vi "EX 10-2_TempControl.vi"() -> ()   [LabVIEW 2010]
uses:
  <vilib>/LabVIEW Interface for Arduino/Type Defs/Pin Mode.ctl
  <vilib>/LabVIEW Interface for Arduino/Type Defs/Board Type.ctl
  <vilib>/LabVIEW Interface for Arduino/Type Defs/Connection Type.ctl
  <vilib>/LabVIEW Interface for Arduino/LabVIEW Interface for Arduino.lvlib
panel:
  in  "手動     /    自動":bool
  in  "熱敏電阻PIN腳":u8
  in  "Units":enum16{"Celsius", "Fahrenheit", "Kelvin"}(ring)
  out "Temperature":dbl(slide) scale=0.0..100.0
  in  "Paired Resistance (Ohms)":dbl=10000.0
  in  "motor 3":u8(slide) scale=0.0..255.0
  in  "motor 1":u8(slide) scale=0.0..255.0
  in  "motor 2":u8(slide) scale=0.0..255.0
  in  "Heater":bool
  in  "最高溫度":dbl
  in  "最低溫度":dbl
  in  "stop":bool
  in  "風扇3 PIN腳":u8=6 min=2 max=13 step=1
  in  "風扇2 PIN腳":u8=5 min=2 max=13 step=1
  in  "風扇1 PIN腳":u8=3 min=2 max=13 step=1
  in  "加熱片PIN腳":u8
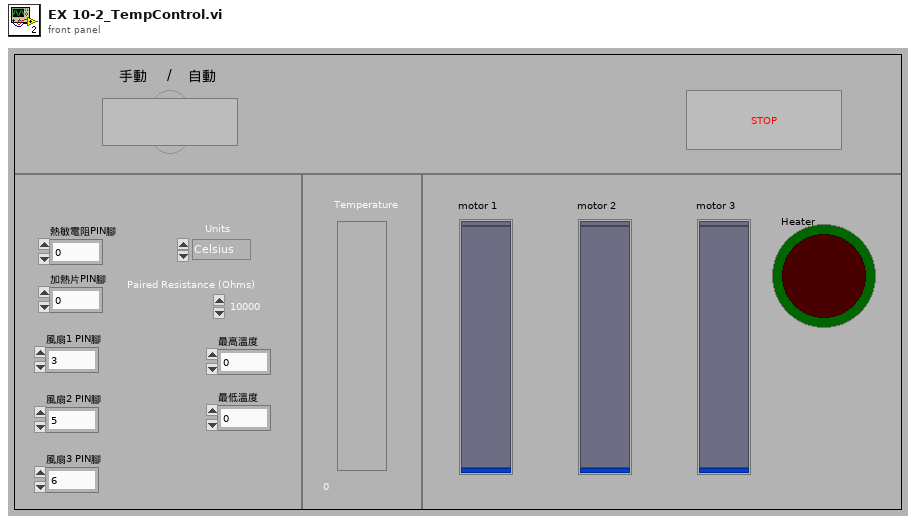
[diagram p1: front panel]
types:
  T1 = typedef "LabVIEW Interface for Arduino.lvlib/Connection Type.ctl" = enum8{"USB / Serial", "XBEE", "BlueSmirf (Bluetooth)"}
  T2 = typedef "LabVIEW Interface for Arduino.lvlib/Board Type.ctl" = enum16{"Uno", "Dimuelanove w/Atmega 328", "Mega 2560"}
  T3 = typedef "LabVIEW Interface for Arduino.lvlib/Pin Mode.ctl" = enum8{"Input", "Output"}
  T4 = typedef "LabVIEW Interface for Arduino.lvlib/Arduino Resource.ctl" = cluster{"VISA resource":refnum<visa-resource-name>, "Board Type":T2, "Connection Type":enum8{"USB / Serial"}, "Bytes Per Packet (15)":u8}
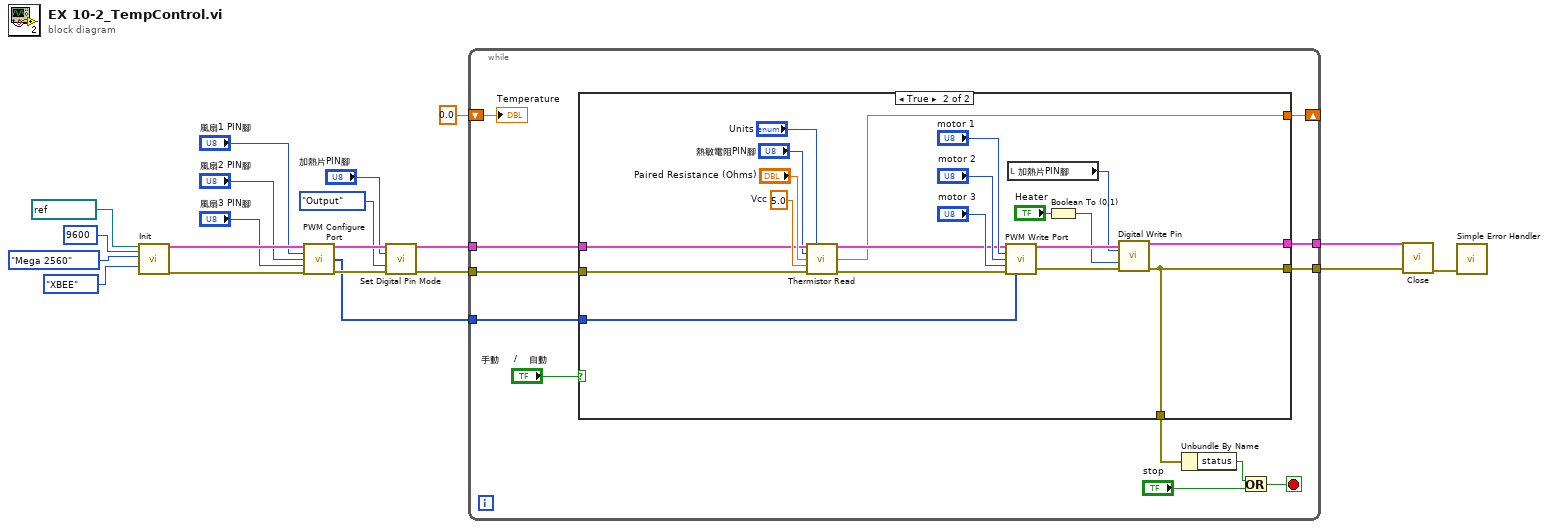
[diagram p0: block diagram]
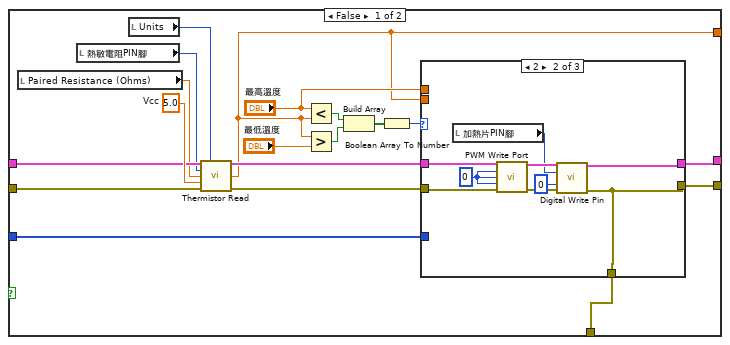
[diagram p2: hidden frame]
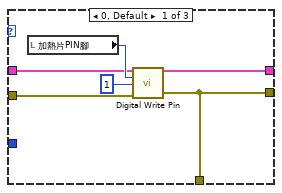
[diagram p3: hidden frame]
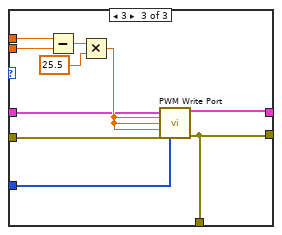
[diagram p4: hidden frame]
diagram:
  n1 = call <vilib>:"Init.vi"("VISA resource"=refnum<visa-resource-name> "COM8", "Baud Rate (115200)"=u32 9600, "Board Type (Uno)"=Board_Type."Mega 2560", "Connection Type (USB/Serial)"=Connection_Type."XBEE") -> ("Arduino Resource"=w19:T4, "error out"=w18:errorcluster)  [unwired: 14 in]
  n2 = call <vilib>:"PWM Configure Port.vi"("Arduino Resource"=w19, "PWM Pin (3)"="風扇1 PIN腳", "PWM Pin (5)"="風扇2 PIN腳", "PWM Pin (6)"="風扇3 PIN腳", "error in"=w18) -> ("Arduino Resource"=w14:T4, "PWM Pins"=w2:u8[], "error out"=w13:errorcluster)  [unwired: 8 in]
  n3 = call <vilib>:"Set Digital Pin Mode.vi"("Arduino Resource"=w14, "Digital I/O Pin"="加熱片PIN腳", "Pin Mode (Input)"=Pin_Mode."Output", "error in"=w13) -> ("Arduino Resource"=w10:T4, "error out"=w9:errorcluster)  [unwired: 10 in]
  n4 = while {
    tunnel: w10 -> [w31]
    tunnel: w9 -> [w30]
    tunnel: [w29] -> w8
    tunnel: [w28] -> w7
    tunnel: w2 -> [w23]
    shift-right: [w21] -> _
    shift-left: 0.0 ("Temperature") -> [w22]
    stop <- w24 stop-if-true
    n5 = case shown="True" "手動     /    自動" {
      tunnel: w31 -> [w50 w93]
      tunnel: w30 -> [w49 w92]
      tunnel: [w38 w80] -> w29
      tunnel: [w36 w79] -> w27
      tunnel: [w37 w79] -> w28
      tunnel: w23 -> [w35 w78]
      tunnel: [w33 w77] -> w21
      frame False {
        w51 = 5.0  # Vcc
        n6 = local read "Paired Resistance (Ohms)"() -> (w46:dbl)
        n7 = local read "熱敏電阻PIN腳"() -> (w47:u8)
        n8 = local read "Units"() -> (w48:enum16{"Celsius", "Fahrenheit", "Kelvin"})
        n9 = call <vilib>:"Thermistor Read.vi"("Arduino Resource"=w50, "Units (C)"=w48, "Thermistor AI Pin (0)"=w47, "Paired Resistance (10K Ohms)"=w46, "Vcc (5 v)"=w51, "error in"=w49) -> ("Arduino Resource"=w40:T4, "Temperature"=w33:dbl, "error out"=w39:errorcluster)  [unwired: 7 in]
        n10 = Less?(x="最高溫度", y=w33) -> (x < y?=w44:bool)
        n11 = Greater?(x=w33, y="最低溫度") -> (0:w43:bool)
        n12 = Build Array(w44, w43) -> (w42:bool[])
        n13 = Boolean Array To Number(Boolean array=w42) -> (number=w41:u32)
        n14 = case shown="2" w41 {
          tunnel: w40 -> [w55 w61 w73]
          tunnel: w39 -> [w54 w60 w72]
          tunnel: [w53 w59 w71] -> w38
          tunnel: [w52 w58 w67] -> w37
          tunnel: [w52 w58 w67] -> w36
          tunnel: w35 -> [_ _ w70]
          tunnel: "最高溫度" -> [_ _ w69]
          tunnel: w33 -> [_ _ w68]
          frame 0, Default {
            n15 = local read "加熱片PIN腳"() -> (w57:u8)
            n16 = call <vilib>:"Digital Write Pin.vi"("Arduino Resource"=w55, "Digital I/O Pin (0)"=w57, "Value (0)"=u8 1, "error in"=w54) -> ("Arduino Resource"=w53:T4, "error out"=w52:errorcluster)  [unwired: 10 in]
          }
          frame 2 {
            w66 = u8 0 ("PWM 0 (0-255)")
            n17 = local read "加熱片PIN腳"() -> (w63:u8)
            n18 = call <vilib>:"PWM Write Port.vi"("Arduino Resource"=w61, "PWM 0 (0-255)"=w66, "PWM 1 (0-255)"=w66, "PWM 2 (0-255)"=w66, "error in"=w60) -> ("Arduino Resource"=w65:T4, "error out"=w64:errorcluster)  [unwired: 8 in, 1 out]
            n19 = call <vilib>:"Digital Write Pin.vi"("Arduino Resource"=w65, "Digital I/O Pin (0)"=w63, "Value (0)"=u8 0, "error in"=w64) -> ("Arduino Resource"=w59:T4, "error out"=w58:errorcluster)  [unwired: 10 in]
          }
          frame 3 {
            n20 = Subtract(x=w69, y=w68) -> (x-y=w74:dbl)
            n21 = Multiply(x=w74, y=25.5) -> (x*y=w76:dbl)
            n22 = call <vilib>:"PWM Write Port.vi"("Arduino Resource"=w73, "PWM Pins"=w70, "PWM 0 (0-255)"=w76, "PWM 1 (0-255)"=w76, "PWM 2 (0-255)"=w76, "error in"=w72) -> ("Arduino Resource"=w71:T4, "error out"=w67:errorcluster)  [unwired: 7 in, 1 out]
          }
        }
      }
      frame True {
        w94 = 5.0  # Vcc
        n23 = call <vilib>:"Thermistor Read.vi"("Arduino Resource"=w93, "Units (C)"="Units", "Thermistor AI Pin (0)"="熱敏電阻PIN腳", "Paired Resistance (10K Ohms)"="Paired Resistance (Ohms)", "Vcc (5 v)"=w94, "error in"=w92) -> ("Arduino Resource"=w87:T4, "Temperature"=w77:dbl, "error out"=w86:errorcluster)  [unwired: 7 in]
        n24 = call <vilib>:"PWM Write Port.vi"("Arduino Resource"=w87, "PWM Pins"=w78, "PWM 0 (0-255)"="motor 1", "PWM 1 (0-255)"="motor 2", "PWM 2 (0-255)"="motor 3", "error in"=w86) -> ("Arduino Resource"=w85:T4, "error out"=w84:errorcluster)  [unwired: 7 in, 1 out]
        n25 = local read "加熱片PIN腳"() -> (w83:u8)
        n26 = Boolean To (0,1)(Boolean="Heater") -> (0, 1=w81:i16)
        n27 = call <vilib>:"Digital Write Pin.vi"("Arduino Resource"=w85, "Digital I/O Pin (0)"=w83, "Value (0)"=w81, "error in"=w84) -> ("Arduino Resource"=w80:T4, "error out"=w79:errorcluster)  [unwired: 10 in]
      }
    }
    n28 = Unbundle By Name(w27) -> ("status"=w26:bool)
    n29 = Or(x=w26, y="stop") -> (x .or. y?=w24:bool)
    "Temperature" <- w22
  }
  n30 = call <vilib>:"Close.vi"("Arduino Resource"=w8, "error in"=w7) -> ("error out"=w20:errorcluster)  [unwired: 13 in]
  n31 = call <vilib>:"Simple Error Handler.vi"("error in (no error)"=w20) -> ()  [unwired: 4 in, 5 out]
